vi "Configure and start movement.vi"(7 "Final wavelength":dbl, 8 "error in (no error)":errorcluster, 9 "Initial wavelength":dbl, 10 "Mono Mod ID":i32, 11 "Speed":dbl) -> (0 "error out":errorcluster)   [LabVIEW 2020]
uses:
  Monochromator/Libraries/Monochromator/Monochromator.lvlib
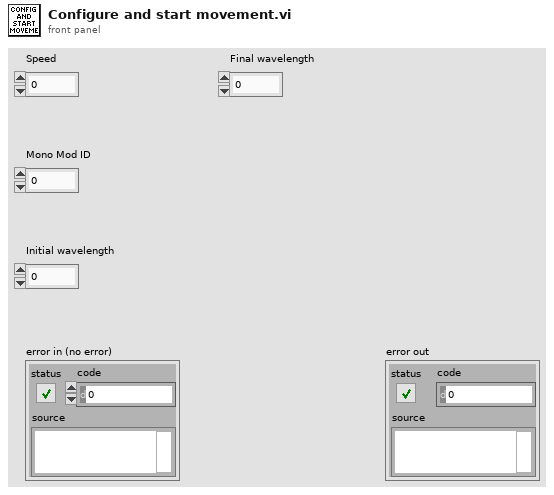
[diagram p1: front panel]
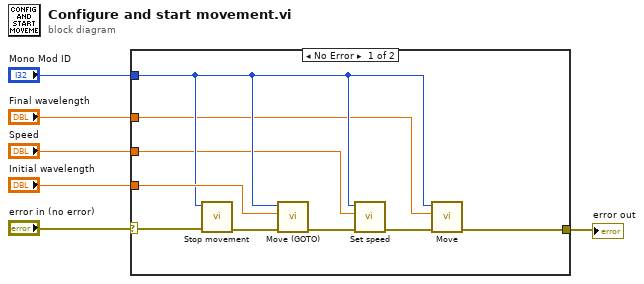
[diagram p0: block diagram]
diagram:
  n1 = case shown="No Error" "error in (no error)" {
    selector: "error in (no error)" -> [w8 w16]
    tunnel: "Initial wavelength" -> [w14 _]
    tunnel: "Mono Mod ID" -> [w13 _]
    tunnel: [w11 w16] -> w4
    tunnel: "Speed" -> [w9 _]
    tunnel: "Final wavelength" -> [w7 _]
    frame No Error {
      n2 = call "Stop movement.vi"("error in"=w8, "Module ID"=w13) -> ("error out"=w12:errorcluster)  [unwired: 9 in]
      n3 = call "Move (GOTO).vi"("error in"=w12, "Position"=w14, "Module ID"=w13) -> ("error out"=w15:errorcluster)  [unwired: 8 in]
      n4 = call "Set speed.vi"("error in"=w15, "nm/min"=w9, "Module ID"=w13) -> ("error out"=w10:errorcluster)  [unwired: 8 in]
      n5 = call "Move.vi"("error in"=w10, "Wavelength"=w7, "Module ID"=w13) -> ("error out"=w11:errorcluster)  [unwired: 8 in]
    }
    frame Error {
    }
  }
  "error out" <- w4
